vi "zad3.vi"() -> ()   [LabVIEW 2018]
panel:
  out "data out":string
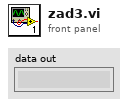
[diagram p1: front panel]
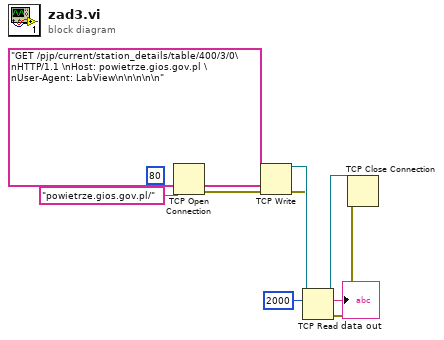
[diagram p0: block diagram]
diagram:
  n1 = TCP Open Connection(address="powietrze.gios.gov.pl/", remote port or service name=u16 80) -> (connection ID=w9:refnum<k5>, error out=w8:errorcluster)  [unwired: 3 in]
  n2 = TCP Write(connection ID=w9, data in="GET /pjp/current/station_details/table/400/3/0\nHTTP/1.1 \nHost: powietrze.gios.gov.pl \nUser-Agent: LabView\n\n\n\n\n", error in (no error)=w8) -> (connection ID out=w5:refnum<k5>, error out=w4:errorcluster)  [unwired: 1 in, 1 out]
  n3 = TCP Read(connection ID=w5, bytes to read=2000, error in (no error)=w4) -> (connection ID out=w2:refnum<k5>, data out=→"data out":string, error out=w1:errorcluster)  [unwired: 2 in]
  n4 = TCP Close Connection(connection ID=w2, error in (no error)=w1) -> ()  [unwired: 1 in, 2 out]
